vi "APD data extraction.vi"(0 "Data":u32[](array[numeric]), 1 "Number of APD's":u8, 2 "APD integration time (s)":dbl, 3 "APD Ave N":dbl, 4 "APD Disp. Downsample":dbl, 5 "APD Disp. Scale":dbl, 8 "Time Stamp":timestamp) -> (6 "Output cluster":T2, 7 "Output Data":T1, 9 "Output waveform":waveform(dbl)[](array[waveform]), 10 "APD Display period (s)":dbl)   [LabVIEW 2014]
uses:
  <vilib>/Analysis/NI_AALBase.lvlib
panel:
  in  "APD Integration Time (s)":dbl=0.001 caption="Integration Time (s)"
  in  "Initialize Cluster":T2
  out "APD 1 Rate (Hz)":dbl format="%#_3p"
  out "Int. Time (s)":dbl=6.0
  out "Rate sigma (Hz)":dbl caption="Sigma (Hz)" format="%0.2f"
  out "Sigma/Mean":dbl=nan format="%#_2g"
  out "APD 2 Rate (Hz)":dbl format="%#_3p"
  out "Rate sigma (Hz)":dbl caption="Sigma (Hz)" format="%0.2f"
  out "Sigma/Mean":dbl=nan format="%#_2g"
  out "APD 3 Rate (Hz)":dbl format="%#_3p"
  out "Rate sigma (Hz)":dbl caption="Sigma (Hz)" format="%0.2f"
  out "Sigma/Mean":dbl=nan format="%#_2g"
types:
  T1 = cluster{"APD 1":u32[], "APD 2":u32[], "APD 3":u32[]}
  T2 = cluster{"APD 1 Rate (Hz)":dbl, "APD 2 Rate (Hz)":dbl, "APD 3 Rate (Hz)":dbl, "Sigma/Mean 1":dbl, "Int Time (s)":dbl, "Sigma 1":dbl, "Sigma 2":dbl, "Sigma 3":dbl, "Sigma/Mean 2":dbl, "Sigma/Mean 3":dbl}
  T3 = enum16{"empty", "write", "read oldest (queue)", "read newest (stack)", "read all"}
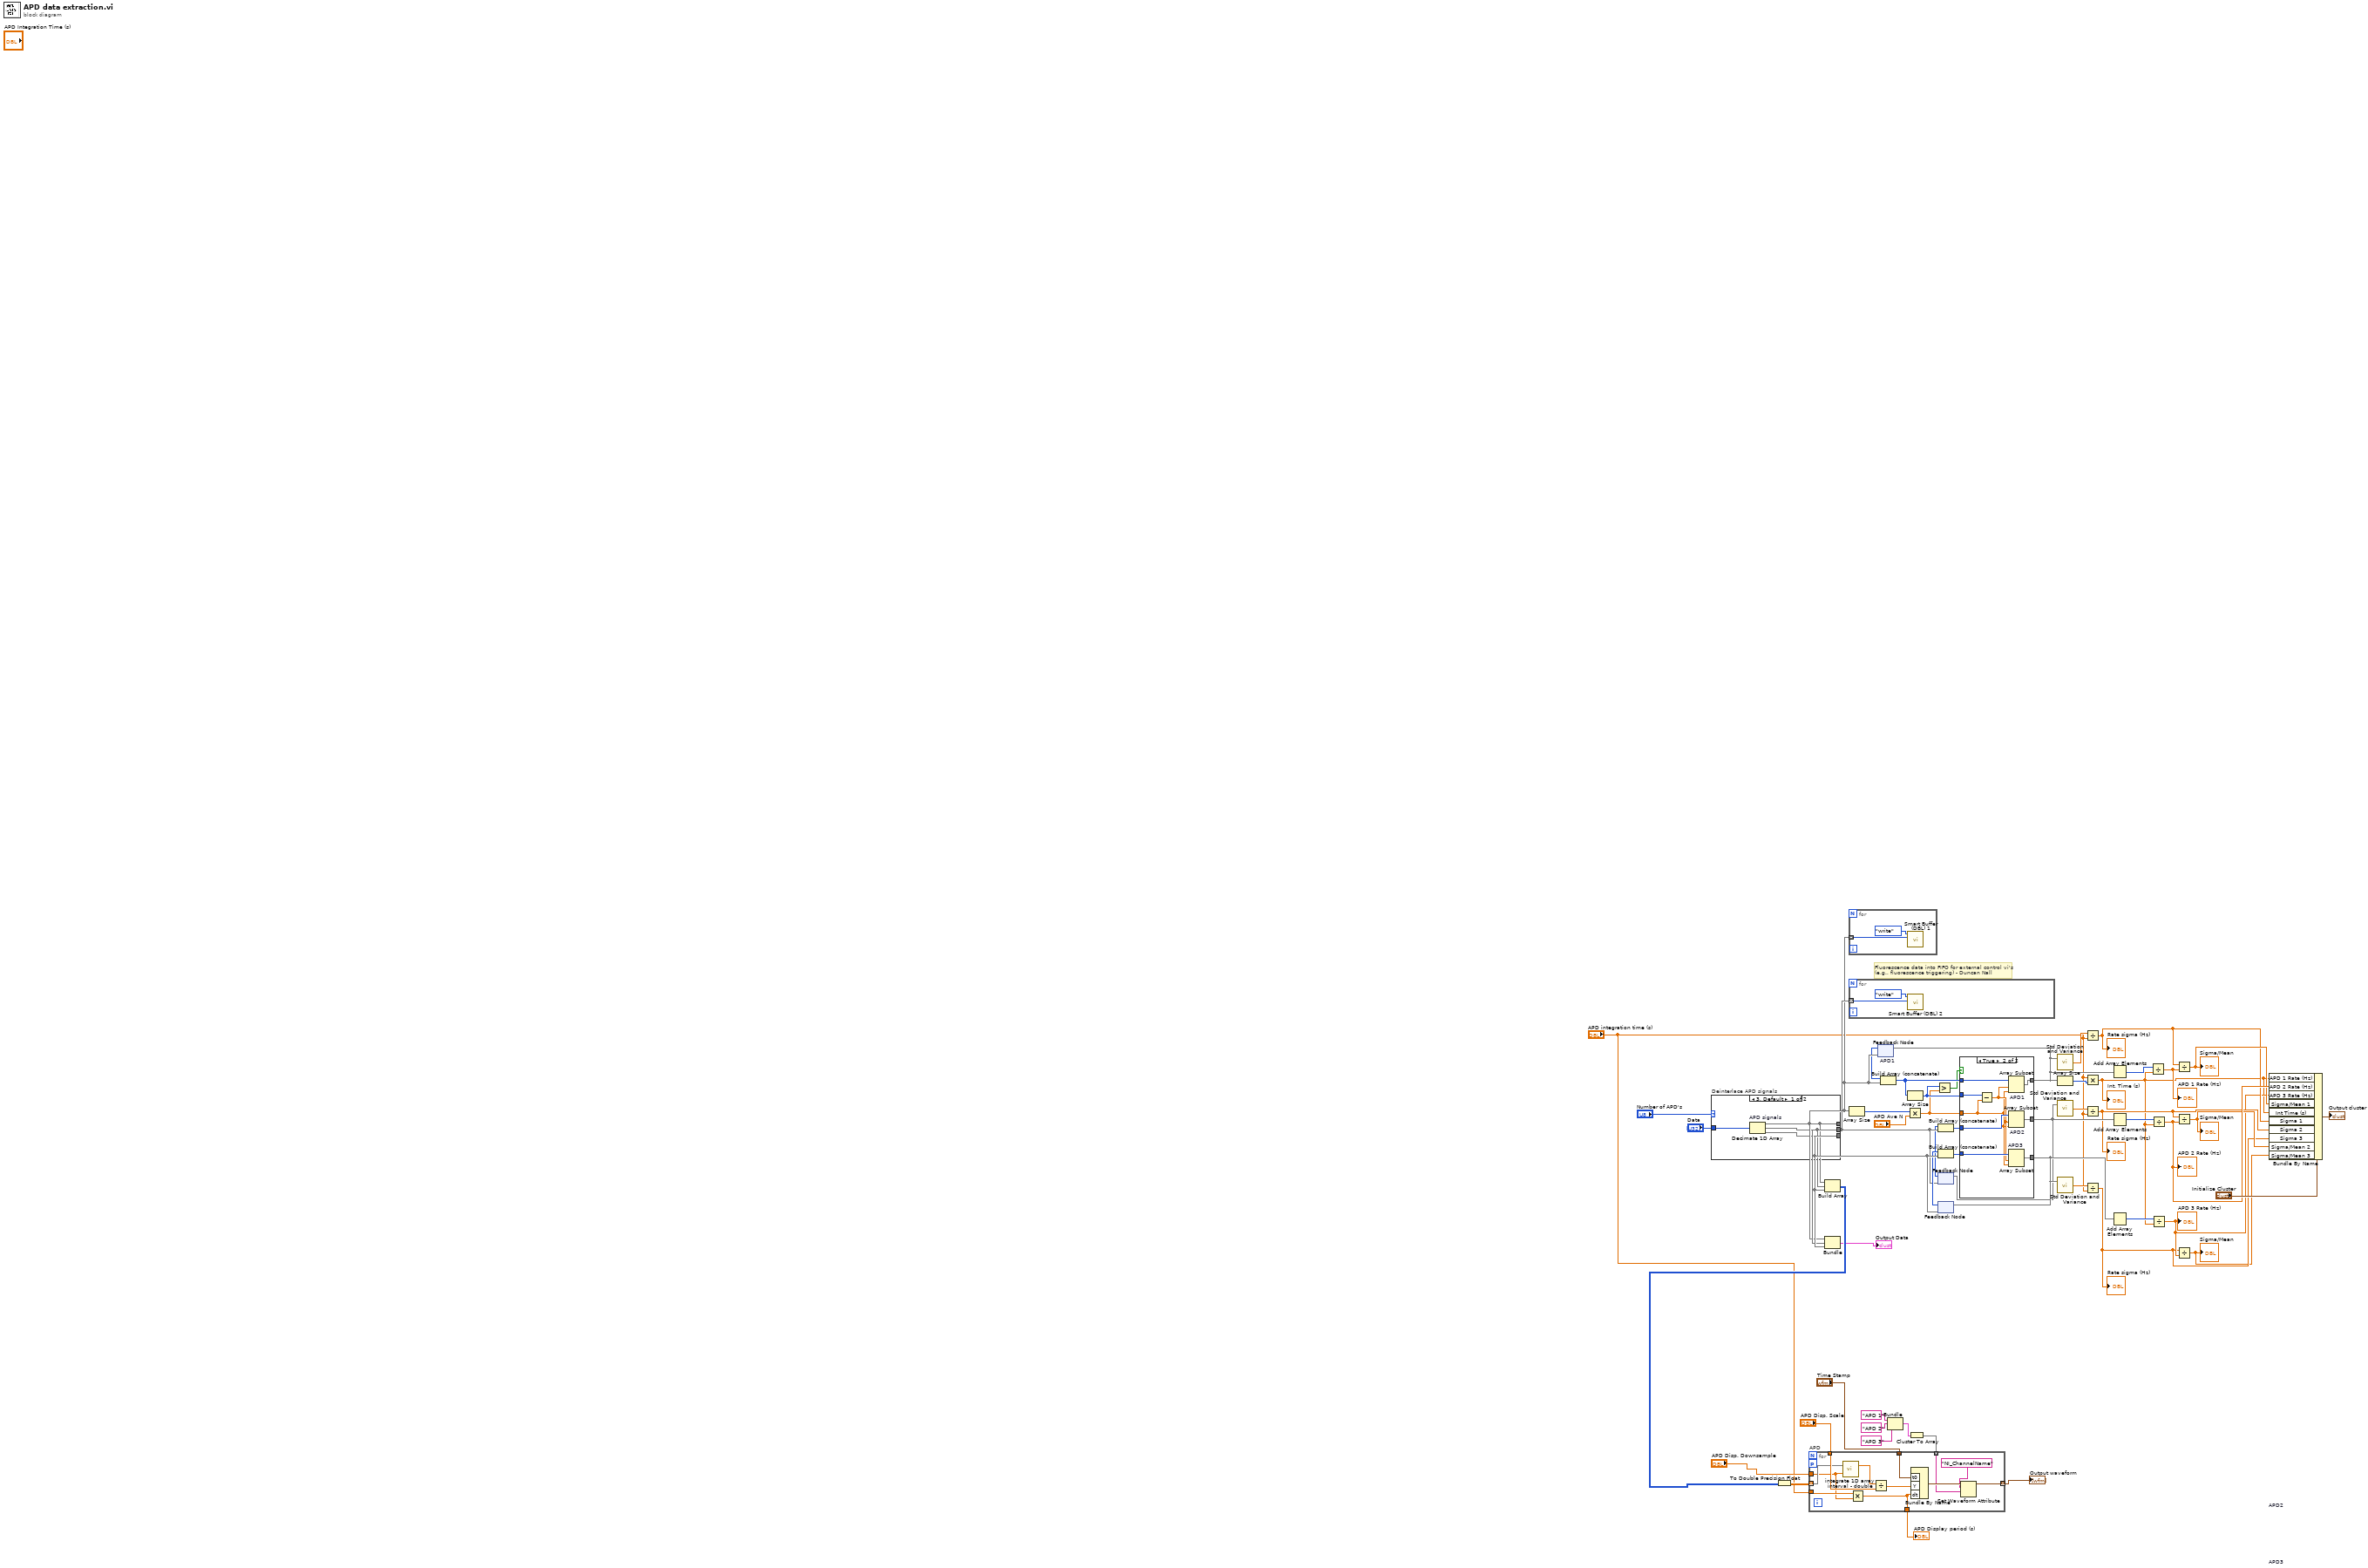
[diagram p0: block diagram]
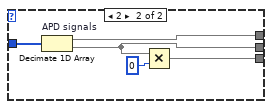
[diagram p2: hidden frame]
diagram:
  # "Fluorescence data into FIFO for external control vi's\n(e.g., fluorescence triggering) - Duncan Nall"
  n1 = case "Deinterlace APD signals" shown="3, Default" "Number of APD's" {
    tunnel: [w55 w61] -> w48
    tunnel: "Data" -> [w56 w60]
    tunnel: [w54 w59] -> w49
    tunnel: [w53 w57] -> w51
    frame 3, Default {
      n2 = Decimate 1D Array "APD signals"(w56) -> (w55:u32[], w54:u32[], w53:u32[])
    }
    frame 2 {
      n3 = Decimate 1D Array "APD signals"(w60) -> (w61:u32[], w59:u32[])
      n4 = Multiply(x=w59, y=u32 0) -> (x*y=w57:u32[])
    }
  }
  n5 = Build Array(w48, w49, w51) -> (w6:u32[][])
  n6 = To Double Precision Float(number=w6) -> (double precision float=w13:dbl[][])
  n7 = Bundle(w48, w49, w51) -> (→"Output Data":cluster{u32[], u32[], u32[]})  [unwired: 1 in]
  n8 = for {
    tunnel: w48 -> [w62] mode=indexing
    n9 = call "Smart Buffer (DBL) 1.vi"("new element [write]"=w62, "mode"=T3."write") -> ()  [unwired: 4 in, 6 out]
  }
  n10 = for {
    tunnel: w49 -> [w65] mode=indexing
    n11 = call "Smart Buffer (DBL) 2.vi"("new element [write]"=w65, "mode"=T3."write") -> ()  [unwired: 4 in, 6 out]
  }
  n12 = Array Size(array=w48) -> (size(s)=w33:i32)
  n13 = feedback #1 "APD1"(w48) -> (w30:u32[])
  n14 = Build Array (concatenate)(w30, w48) -> (w32:u32[])
  n15 = Bundle("APD 1", "APD 2", "APD 3") -> (w9:cluster{string, string, string})  [unwired: 1 out]
  n16 = Multiply(x=w33, y="APD Ave N") -> (x*y=w34:dbl)
  n17 = Array Size(array=w32) -> (size(s)=w35:i32)
  n18 = Cluster To Array(cluster=w9) -> (array=w12:string[])
  n19 = for "APD" {
    tunnel: w13 -> [w70] mode=indexing
    tunnel: "APD integration time (s)" -> [w77]
    tunnel: [w73] -> w2 mode=indexing
    tunnel: "APD Disp. Scale" -> [w74]
    tunnel: w12 -> [w72] mode=indexing
    tunnel: "APD Disp. Downsample" -> [w68]
    tunnel: [w71] -> w1
    workers-P: _ -> [_]
    tunnel: "Time Stamp" -> [w67]
    n20 = call "integrate 1D array interval - double.vi"("Ave N"=w68, "Array In"=w70) -> ("Array Out"=w69:dbl[])  [unwired: 1 out]
    n21 = Multiply(x=w77, y=w68) -> (x*y=w71:dbl)
    n22 = Divide(x=w69, y=w74) -> (x/y=w75:dbl[])
    n23 = Bundle By Name("t0"=w67, "Y"=w75, "dt"=w71) -> (w76:waveform(dbl))  [unwired: 1 out]
    n24 = Set Waveform Attribute(5:w72, 6:"NI_ChannelName" ("name"), 7:w76) -> (3:w73:waveform(dbl))  [unwired: 1 in, 2 out]
  }
  "Output waveform" <- w2
  "APD Display period (s)" <- w1
  n25 = Greater?(x=w35, y=w34) -> (0:w31:bool)
  n26 = feedback #2 "APD2"(w49) -> (w40:u32[])
  n27 = Build Array (concatenate)(w40, w49) -> (w41:u32[])
  n28 = feedback #3 "APD3"(w51) -> (w50:u32[])
  n29 = Build Array (concatenate)(w50, w51) -> (w52:u32[])
  n30 = case shown="True" w31 {
    tunnel: w32 -> [w80 w89]
    tunnel: [w80 w87] -> w37
    tunnel: w34 -> [_ w82]
    tunnel: w35 -> [_ w88]
    tunnel: w41 -> [w79 w86]
    tunnel: [w79 w85] -> w43
    tunnel: w52 -> [w78 w84]
    tunnel: [w78 w81] -> w47
    frame False {
    }
    frame True {
      n31 = Subtract(x=w88, y=w82) -> (x-y=w83:dbl)
      n32 = Array Subset "APD1"(array=w89, index=w83, length=w82) -> (w87:u32[])
      n33 = Array Subset "APD2"(array=w86, index=w83, length=w82) -> (w85:u32[])
      n34 = Array Subset "APD3"(array=w84, index=w83, length=w82) -> (w81:u32[])
    }
  }
  n35 = feedback-in #1(w37) -> ()
  n36 = feedback-in #2(w43) -> ()
  n37 = feedback-in #3(w47) -> ()
  n38 = call <vilib>:"Std Deviation and Variance.vi"("X"=w37) -> ("standard deviation"=w38:dbl)  [unwired: 1 in, 2 out]
  n39 = Array Size(array=w37) -> (size(s)=w36:i32)
  n40 = call <vilib>:"Std Deviation and Variance.vi"("X"=w43) -> ("standard deviation"=w44:dbl)  [unwired: 1 in, 2 out]
  n41 = call <vilib>:"Std Deviation and Variance.vi"("X"=w47) -> ("standard deviation"=w46:dbl)  [unwired: 1 in, 2 out]
  n42 = Divide(x=w38, y="APD integration time (s)") -> (x/y=w20:dbl)
  "Rate sigma (Hz)" <- w20
  n43 = Multiply(x="APD integration time (s)", y=w36) -> (x*y=w16:dbl)
  "Int. Time (s)" <- w16
  n44 = Divide(x=w44, y="APD integration time (s)") -> (x/y=w23:dbl)
  "Rate sigma (Hz)" <- w23
  n45 = Divide(x=w46, y="APD integration time (s)") -> (x/y=w18:dbl)
  "Rate sigma (Hz)" <- w18
  n46 = Add Array Elements(numeric array=w37) -> (sum=w29:u32)
  n47 = Add Array Elements(numeric array=w43) -> (sum=w42:u32)
  n48 = Add Array Elements(numeric array=w47) -> (sum=w45:u32)
  n49 = Divide(x=w29, y=w16) -> (x/y=w39:dbl)
  "APD 1 Rate (Hz)" <- w39
  n50 = Divide(x=w42, y=w16) -> (x/y=w24:dbl)
  "APD 2 Rate (Hz)" <- w24
  n51 = Divide(x=w45, y=w16) -> (x/y=w19:dbl)
  "APD 3 Rate (Hz)" <- w19
  n52 = Divide(x=w20, y=w39) -> (x/y=w21:dbl)
  "Sigma/Mean" <- w21
  n53 = Divide(x=w23, y=w24) -> (x/y=w22:dbl)
  "Sigma/Mean" <- w22
  n54 = Divide(x=w18, y=w19) -> (x/y=w17:dbl)
  "Sigma/Mean" <- w17
  n55 = Bundle By Name(cluster="Initialize Cluster", "APD 1 Rate (Hz)"=w16, "APD 2 Rate (Hz)"=w24, "APD 3 Rate (Hz)"=w19, "Sigma/Mean 1"=w21, "Int Time (s)"=w16, "Sigma 1"=w20, "Sigma 2"=w23, "Sigma 3"=w18, "Sigma/Mean 2"=w22, "Sigma/Mean 3"=w17) -> (→"Output cluster":T2)
